vi "RSNRPZ Advanced Zero.vi"(8 "error in (no error)":errorcluster, 9 "Zeroing (3: Low Frequencies)":i32(ring)=3 items=["Low Frequencies"=3, "High Frequencies"=4], 10 "Channel (1)":i32=1, 11 "VISA session":refnum<visa-resource-name> caption="VISA resource name") -> (0 "error out":errorcluster, 3 "dup VISA session":refnum<visa-resource-name> caption="VISA resource name")   [LabVIEW 2010]
doc: "This VI performs zeroing using the signal at the sensor input. The sensor must be disconnected from all power sources. If the signal at the input considerably deviates from 0 W, an error message is issued and the VI is aborted.\n\nNote(s):\n\n(1) This VI is valid only for NRP-Z81.\n\nRemote-control command(s):\nCAL:ZERO:AUTO LFR | UFR"
uses:
  rsnrpz_32.dll
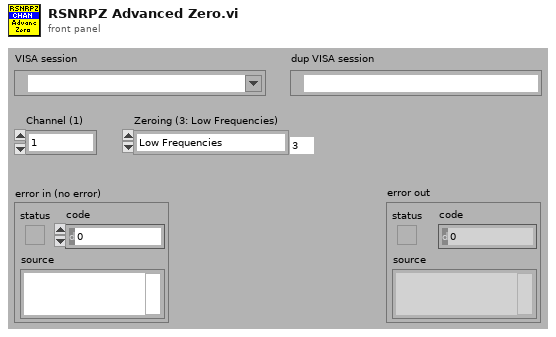
[diagram p1: front panel]
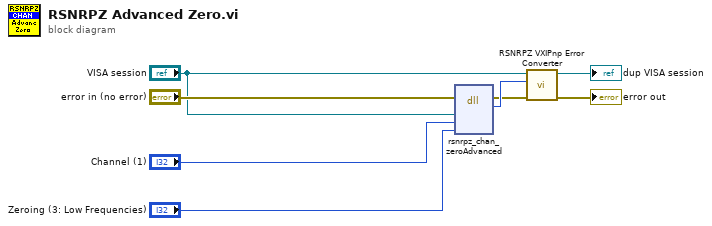
[diagram p0: block diagram]
diagram:
  n1 = dll-call lib="rsnrpz_32.dll" fn="rsnrpz_chan_zeroAdvanced"(error in="error in (no error)", "Instrument Handle"="VISA session", "Channel"="Channel (1)", "Zeroing"="Zeroing (3: Low Frequencies)") -> (error out=w5:errorcluster, "Status"=w8:i32)  [unwired: 5 in, 1 out]
  n2 = call <instrlib>:"RSNRPZ VXIPnp Error Converter.vi"("error in"=w5, "VXIPnp error code"=w8, "VISA session"="VISA session") -> ("error out"=→"error out":errorcluster, "dup VISA session"=→"dup VISA session":refnum<visa-resource-name>)  [unwired: 7 in]
